vi "plcm3GetValue.vi"(6 "Measurement Type":u32(ring) items=["OFF", "1mV range (1mV/A)", "10mV range (10mV/A)", "100mV range (100mV/A)", "Voltage Input"], 7 "Channel":i32, 8 "error in (no error)":errorcluster, 11 "handle in":i16) -> (0 "error out":errorcluster, 2 "Channel Data":dbl, 3 "handle out":i16)   [LabVIEW 2009]
doc: "Calls UsbPt104GetValue for single channel, returns single value."
uses:
  plcm3.dll
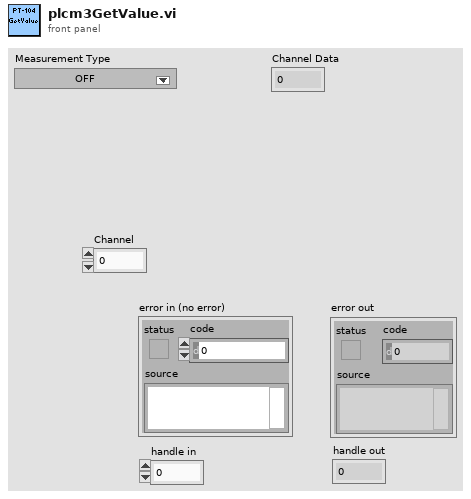
[diagram p1: front panel]
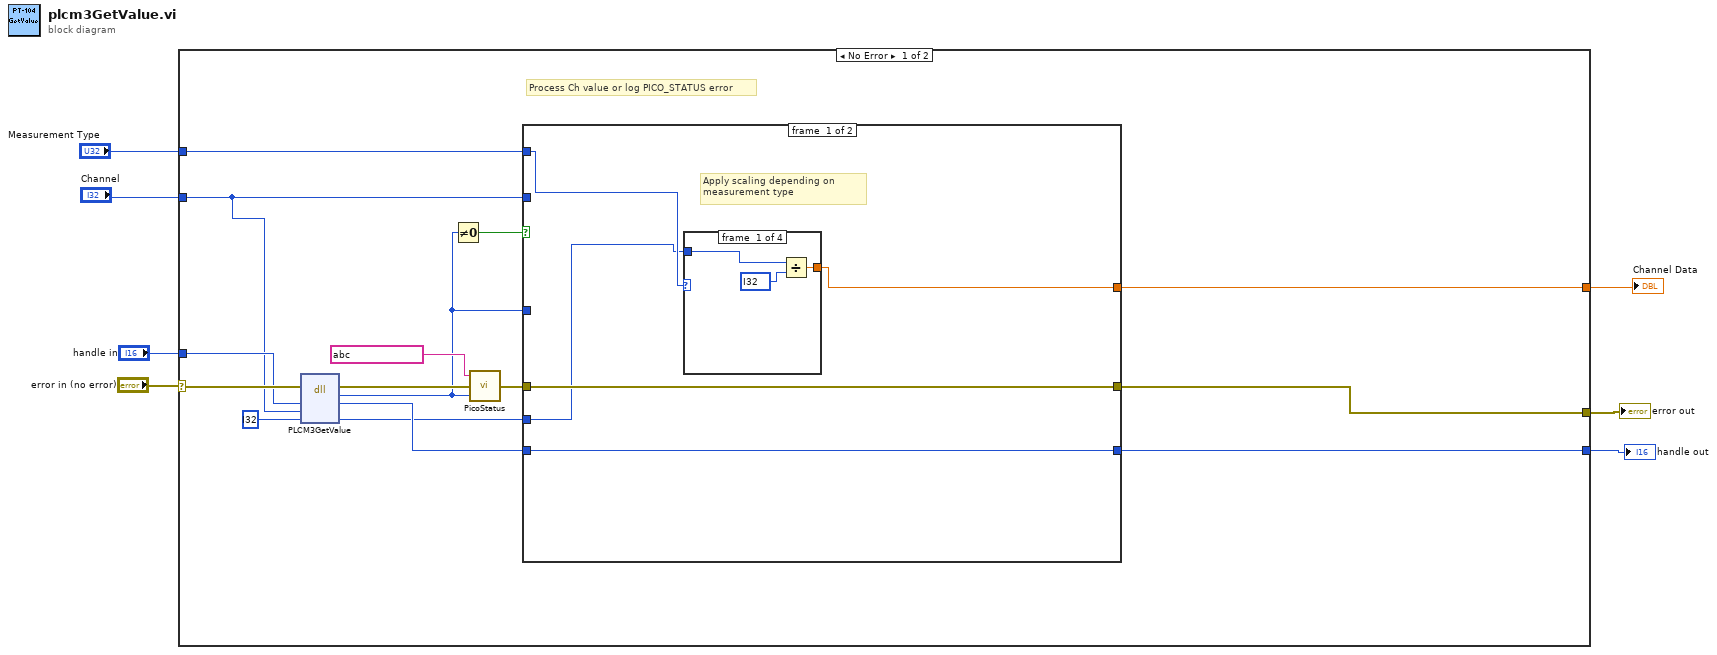
[diagram p0: block diagram]
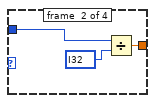
[diagram p2: hidden frame]
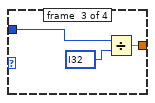
[diagram p3: hidden frame]
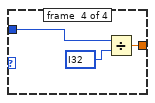
[diagram p4: hidden frame]
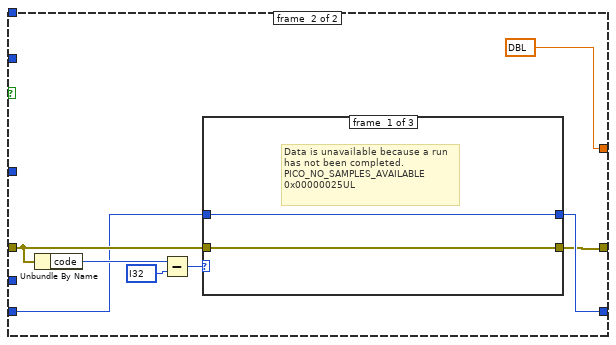
[diagram p5: hidden frame]
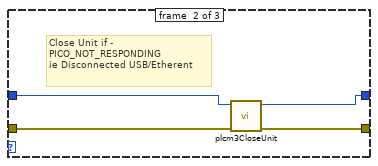
[diagram p6: hidden frame]
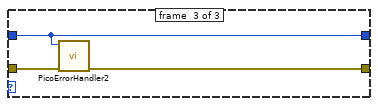
[diagram p7: hidden frame]
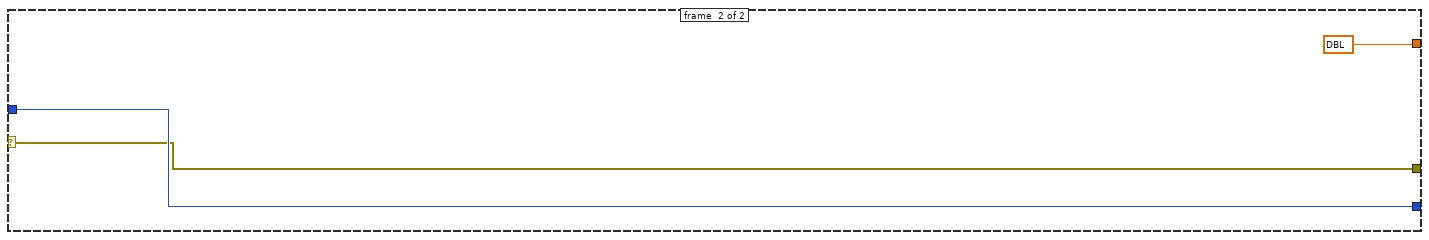
[diagram p8: hidden frame]
diagram:
  n1 = case shown="No Error" "error in (no error)" {
    selector: "error in (no error)" -> [w17 w58]
    tunnel: "handle in" -> [w16 w59]
    tunnel: [w18 w59] -> w7
    tunnel: [w19 w58] -> w6
    tunnel: "Channel" -> [w8 _]
    tunnel: "Measurement Type" -> [w10 _]
    tunnel: [w9 dbl ?] -> w1
    frame #0 {
      # "Process Ch value or log PICO_STATUS error"
      n2 = dll-call lib="PLCM3.dll" fn="PLCM3GetValue"(error in=w17, "handle"=w16, "channel"=w8, "value"=i32 ?) -> (error out=w15:errorcluster, "PICO_STATUS"=w14:u32, "handle"=w13:i16, "value"=w12:i32)  [unwired: 3 in, 1 out]
      n3 = Not Equal To 0?(x=w14) -> (x != 0?=w21:bool)
      n4 = call "PicoStatus.vi"("PICO STATUS"=w14, "error in"=w15, "source"=string ?) -> ("error out"=w20:errorcluster)
      n5 = case shown="True" w21 {
        tunnel: w20 -> [w26 w44]
        tunnel: w8 -> [_ _]
        tunnel: w13 -> [w27 w40]
        tunnel: [w27 w43] -> w18
        tunnel: [w26 w42] -> w19
        tunnel: w14 -> [_ _]
        tunnel: [w23 dbl ?] -> w9
        tunnel: w12 -> [w24 _]
        tunnel: w10 -> [w25 _]
        frame #0 {
          # "Apply scaling depending on \nmeasurement type"
          n6 = case shown="2" w25 {
            tunnel: w24 -> [w29 w32 w35 w38]
            tunnel: [w28 w31 w34 w37] -> w23
            frame #0 {
              n7 = Divide(x=w29, y=i32 ?) -> (x/y=w28:dbl)
            }
            frame #1 {
              n8 = Divide(x=w32, y=i32 ?) -> (x/y=w31:dbl)
            }
            frame #2 {
              n9 = Divide(x=w35, y=i32 ?) -> (x/y=w34:dbl)
            }
            frame #3 {
              n10 = Divide(x=w38, y=i32 ?) -> (x/y=w37:dbl)
            }
          }
        }
        frame #1 {
          n11 = Unbundle By Name(w44) -> ("code"=w47:i32)
          n12 = Subtract(x=w47, y=i32 ?) -> (x-y=w45:i32)
          n13 = case shown="8, Default" w45 {
            tunnel: w40 -> [w49 w50 w55]
            tunnel: w44 -> [w48 w53 w56]
            tunnel: [w49 w51 w55] -> w43
            tunnel: [w48 w52 w54] -> w42
            frame #0 {
              # "Data is unavailable because a run\nhas not been completed.\nPICO_NO_SAMPLES_AVAILABLE \n0x00000025UL"
            }
            frame #1 {
              # "Close Unit if -\nPICO_NOT_RESPONDING\nie Disconnected USB/Etherent"
              n14 = call "plcm3CloseUnit.vi"("error in (no error)"=w53, "handle in"=w50) -> ("error out"=w52:errorcluster, "handle out"=w51:i16)  [unwired: 8 in]
            }
            frame #2 {
              n15 = call "PicoErrorHandler2.vi"("error in (no error)"=w56, "handle In"=w55) -> ("error out"=w54:errorcluster)  [unwired: 9 in]
            }
          }
        }
      }
    }
    frame #1 {
    }
  }
  "error out" <- w6
  "handle out" <- w7
  "Channel Data" <- w1
